vi "TraverseGetSetups.vi"(2 "Speed Factor":dbl=1.0 min=0.1 max=5.0 format="%.2f", 3 "Traverse Name":string="EnFlo Tunnel", 4 "Home":T2) -> (0 "Channel Properties Out":T1[](array[typedef]) {"Current Pos" format="%.2f"; "Backlash/Eng units" format="%.2f"; "Pulses/rev" format="%.2f"; "Pos Tolerance" format="%.2f"; "Pulses/unit" format="%.2f"; "Acc. Min" format="%.2f"; "Acc. Max" format="%.2f"; "Vel. Min" format="%.2f"; "Vel. Max" format="%.2f"; "Acc. Default" format="%.2f"; "Vel. Default" format="%.2f"}, 1 "Error String":string)   [LabVIEW 2022 SP3]
uses:
  Anemometry/Anemometry Sub Vis/Controls/Home.ctl
  ~subVIs/DriveConfigGlobal.vi
  ~subVIs/DriveProperties.ctl
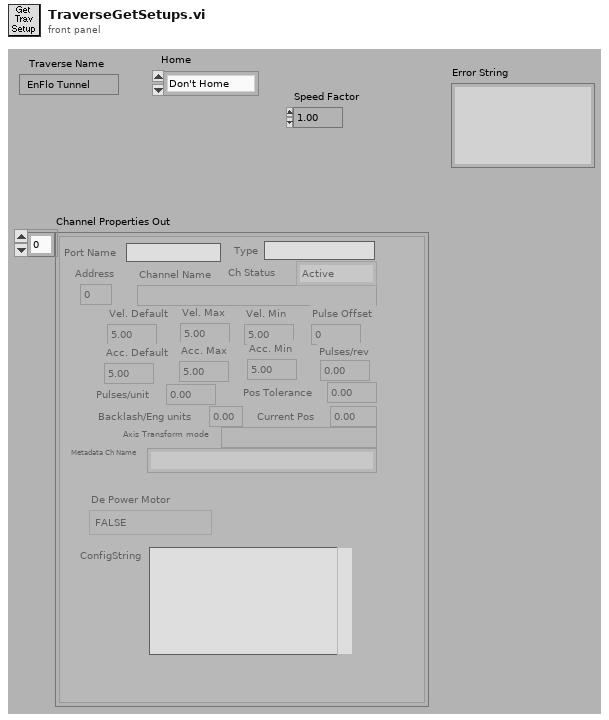
[diagram p1: front panel]
types:
  T1 = typedef "DriveProperties.ctl" = cluster{"Channel Name":string, "Vel. Default":sgl, "Acc. Default":sgl, "Vel. Max":sgl, "Vel. Min":sgl, "Acc. Max":sgl, "Acc. Min":sgl, "Pulses/unit":sgl, "Address":u8, "Pulse Offset":i32, "Pos Tolerance":sgl, "Pulses/rev":sgl, "Backlash/Eng units":sgl, "Current Pos":sgl, "Ch Status":enum16{"Active", "Offline", "Simulate"}, "Port Name":string, "Axis Transform mode":string, "Metadata Ch Name":string, "Type":string, "De Power Motor":enum16{"TRUE", "FALSE"}, "ConfigString":string}
  T2 = typedef "Home.ctl" = enum16{"Don't Home", "Home  +X", "Home  -X", "Home  +Y", "Home  -Y", "Home  +Z", "Home  -Z"}
  T3 = enum16{"Load setup from excel file", "Save setup to excel file"}
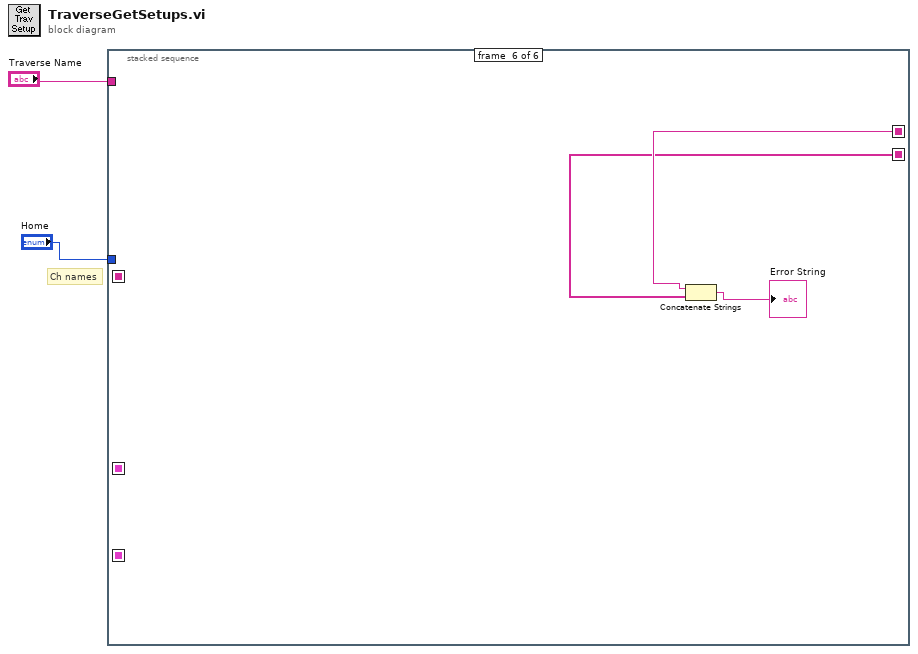
[diagram p0: block diagram]
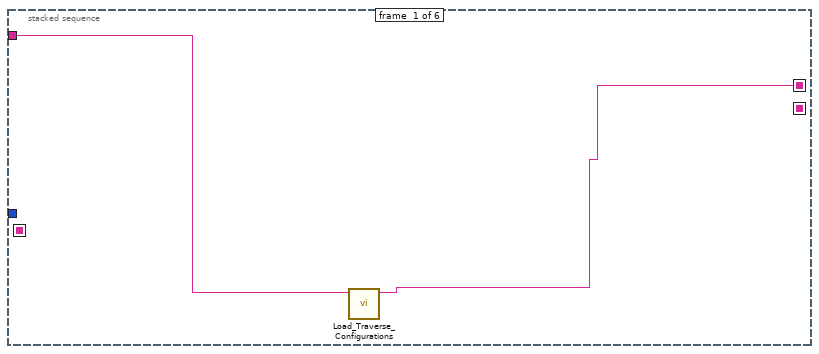
[diagram p2: hidden frame]
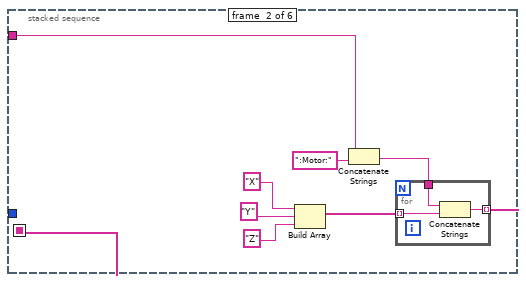
[diagram p3: hidden frame]
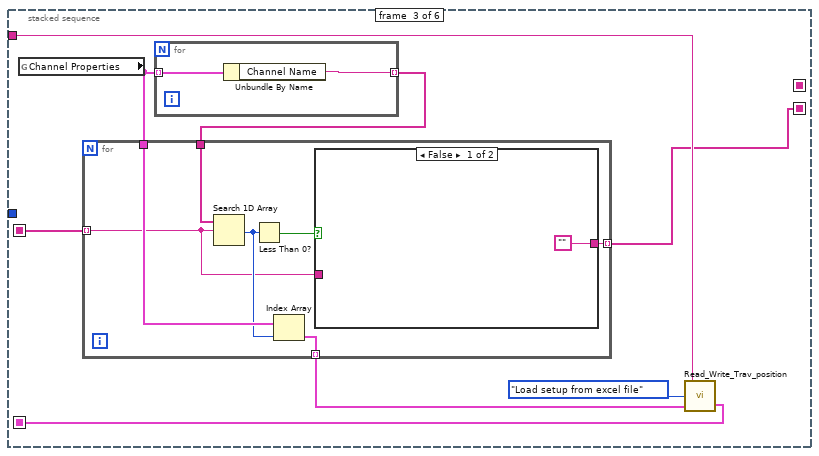
[diagram p4: hidden frame]
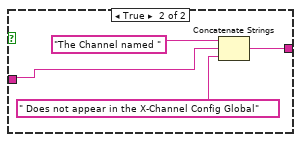
[diagram p5: hidden frame]
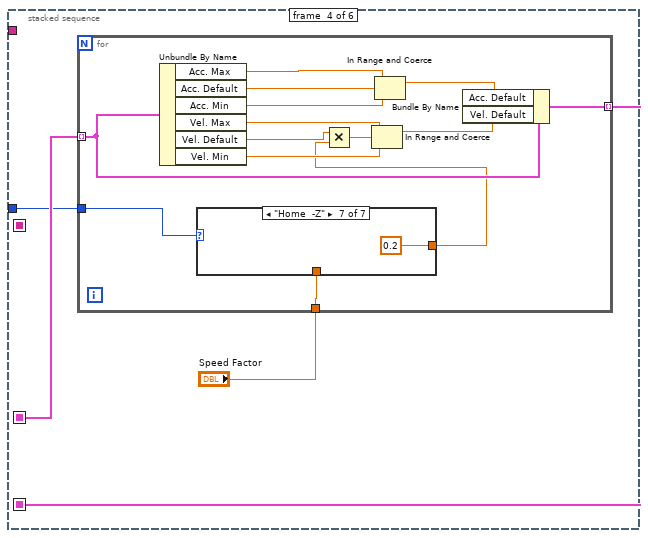
[diagram p6: hidden frame]
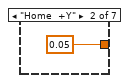
[diagram p8: hidden frame]
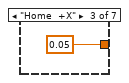
[diagram p9: hidden frame]
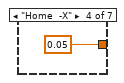
[diagram p10: hidden frame]
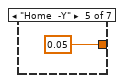
[diagram p11: hidden frame]
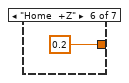
[diagram p12: hidden frame]
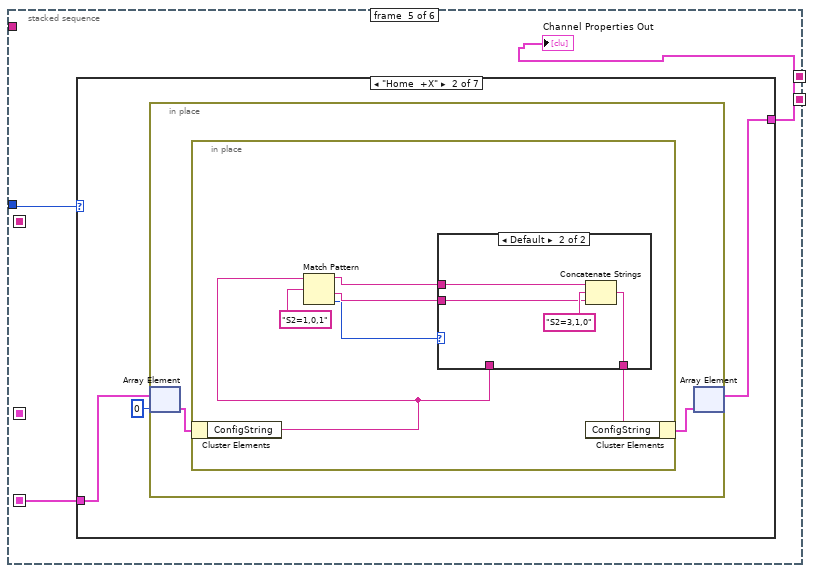
[diagram p13: hidden frame]
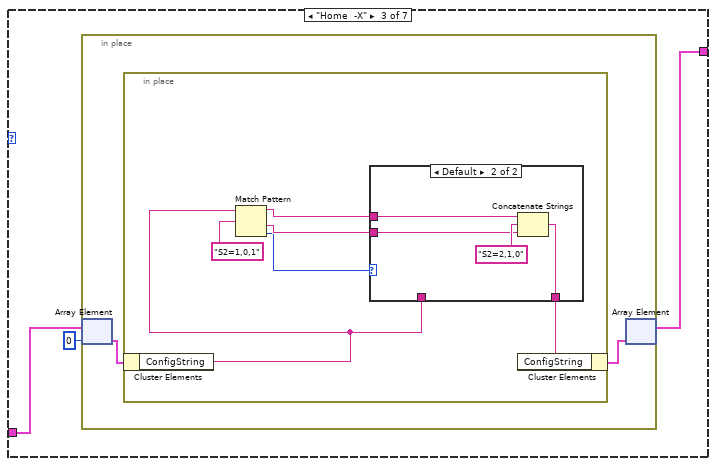
[diagram p16: hidden frame]
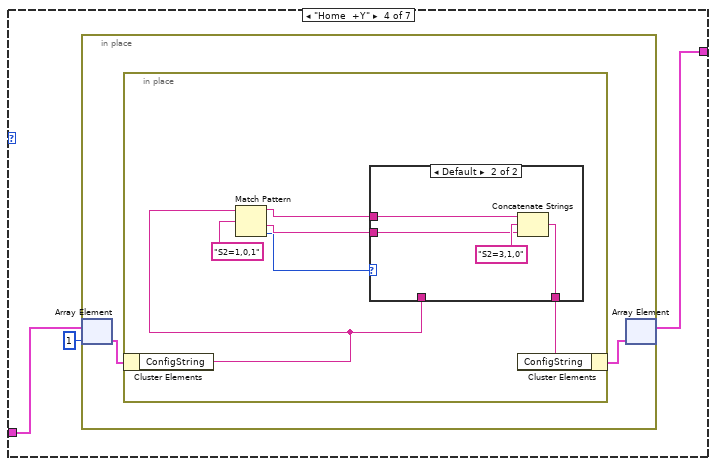
[diagram p18: hidden frame]
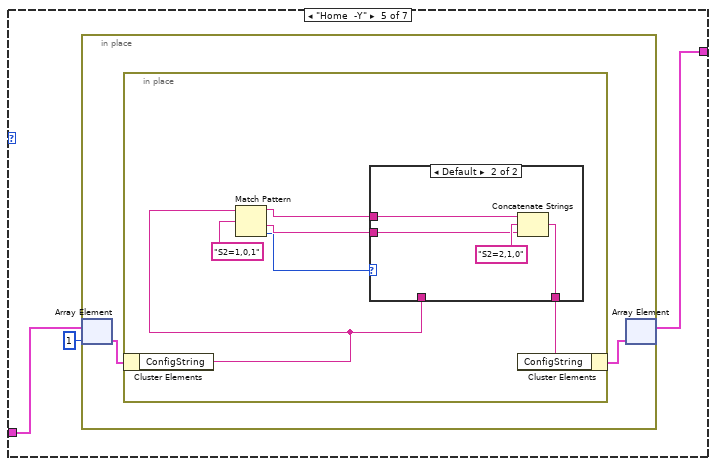
[diagram p20: hidden frame]
diagram:
  # "Ch names"
  n1 = stacked-sequence {
    seq-local: [_ w10 _ _ _ _] -> [_ _ w22 _ _ _]
    seq-local: [_ _ w19 _ _ _] -> [_ _ _ w41 _ _]
    seq-local: [_ _ _ w38 _ _] -> [_ _ _ _ w64 _]
    seq-local: [w3 _ _ _ _ _] -> [_ _ _ _ _ w165]
    seq-local: [_ _ w16 _ _ _] -> [_ _ _ _ _ w164]
    tunnel: "Traverse Name" -> [w4 w8 w18 _ _ _]
    tunnel: "Home" -> [_ _ _ w39 w65 _]
    frame #0 {
      n2 = call "Load_Traverse_Configurations.vi"("Traverse Name"=w4) -> ("Error String"=w3:string)  [unwired: 10 in]
    }
    frame #1 {
      n3 = Build Array("X", "Y", "Z") -> (w11:string[])
      n4 = Concatenate Strings(w8, ":Motor:") -> (w9:string)
      n5 = for {
        tunnel: w11 -> [w15] mode=indexing
        tunnel: [w13] -> w10 mode=indexing
        tunnel: w9 -> [w14]
        n6 = Concatenate Strings(w14, w15) -> (w13:string)
      }
    }
    frame #2 {
      n7 = global read "DriveConfigGlobal.vi" "Channel Properties"() -> (w17:T1[])
      n8 = for {
        tunnel: w17 -> [w37] mode=indexing
        tunnel: [w36] -> w23 mode=indexing
        n9 = Unbundle By Name(w37) -> ("Channel Name"=w36:string)
      }
      n10 = for {
        tunnel: w23 -> [w30]
        tunnel: w17 -> [w28]
        tunnel: [w26] -> w21 mode=indexing
        tunnel: w22 -> [w25] mode=indexing
        tunnel: [w24] -> w16 mode=indexing
        n11 = Search 1D Array(1D array=w30, element=w25) -> (index of element=w27:i32)  [unwired: 1 out]
        n12 = Less Than 0?(x=w27) -> (x < 0?=w29:bool)
        n13 = Index Array(array=w28, index=w27) -> (element=w26:T1)
        n14 = case shown="False" w29 {
          tunnel: w25 -> [_ w34]
          tunnel: ["" w32] -> w24
          frame False {
          }
          frame True {
            n15 = Concatenate Strings("The Channel named " ("message"), w34, " Does not appear in the X-Channel Config Global" ("Input 3")) -> (w32:string)
          }
        }
      }
      n16 = call "Read_Write_Trav_position.vi"("Channel Properties"=w21, "Mode"=T3."Load setup from excel file", "Traverse Name"=w18) -> ("Channel Properties Out"=w19:T1[])  [unwired: 1 out]
    }
    frame #3 {
      n17 = for {
        tunnel: w41 -> [w53] mode=indexing
        tunnel: "Speed Factor" -> [w45]
        tunnel: [w51] -> w38 mode=indexing
        tunnel: w39 -> [w43]
        n18 = Unbundle By Name(w53) -> ("Acc. Max"=w49:sgl, "Acc. Default"=w42:sgl, "Acc. Min"=w48:sgl, "Vel. Max"=w52:sgl, "Vel. Default"=w46:sgl, "Vel. Min"=w55:sgl)
        n19 = case shown="\"Home  -Z\"" w43 {
          tunnel: [w56 0.05 ("Speed Factor") 0.05 ("Speed Factor") 0.05 ("Speed Factor") 0.05 ("Speed Factor") 0.2 ("Speed Factor") 0.2 ("Speed Factor")] -> w44
          tunnel: w45 -> [w56 _ _ _ _ _ _]
          frame "Don't Home" {
          }
          frame "Home  +Y" {
          }
          frame "Home  +X" {
          }
          frame "Home  -X" {
          }
          frame "Home  -Y" {
          }
          frame "Home  +Z" {
          }
          frame "Home  -Z" {
          }
        }
        n20 = Multiply(x=w46, y=w44) -> (x*y=w54:dbl)
        n21 = In Range and Coerce(upper limit=w52, x=w54, lower limit=w55) -> (coerced(x)=w50:dbl)  [unwired: 1 out]
        n22 = In Range and Coerce(upper limit=w49, x=w42, lower limit=w48) -> (coerced(x)=w47:sgl)  [unwired: 1 out]
        n23 = Bundle By Name(cluster=w53, "Acc. Default"=w47, "Vel. Default"=w50) -> (w51:T1)
      }
    }
    frame #4 {
      n24 = case shown="\"Home  +X\"" w65 {
        tunnel: w64 -> [w66 w69 w85 w101 w117 w133 w149]
        tunnel: [w66 w67 w83 w99 w115 w131 w147] -> w63
        frame "Don't Home" {
        }
        frame "Home  +X" {
          n25 = in-place {
            n26 = in-place-array #1(w69, 0) -> (w71:T1)
            n27 = in-place {
              n28 = in-place-cluster #2(w71) -> ("ConfigString"=w72:string)
              n29 = Match Pattern(string=w72, regular expression="S2=1,0,1") -> (before substring=w76:string, after substring=w75:string, offset past match=w73:i32)  [unwired: 1 in, 1 out]
              n30 = case shown="Default" w73 {
                tunnel: w76 -> [_ w82]
                tunnel: w75 -> [_ w80]
                tunnel: [w78 w79] -> w74
                tunnel: w72 -> [w78 _]
                frame -1 {
                }
                frame Default {
                  n31 = Concatenate Strings(w82, "S2=3,1,0" ("regular expression"), w80) -> (w79:string)
                }
              }
              n32 = in-place-cluster #2("ConfigString"=w74) -> (w70:T1)
            }
            n33 = in-place-array #1(w70) -> (w67:T1[])  [unwired: 1 out]
          }
        }
        frame "Home  -X" {
          n34 = in-place {
            n35 = in-place-array #3(w85, 0) -> (w87:T1)
            n36 = in-place {
              n37 = in-place-cluster #4(w87) -> ("ConfigString"=w88:string)
              n38 = Match Pattern(string=w88, regular expression="S2=1,0,1") -> (before substring=w92:string, after substring=w91:string, offset past match=w89:i32)  [unwired: 1 in, 1 out]
              n39 = case shown="Default" w89 {
                tunnel: w92 -> [_ w98]
                tunnel: w91 -> [_ w96]
                tunnel: [w94 w95] -> w90
                tunnel: w88 -> [w94 _]
                frame -1 {
                }
                frame Default {
                  n40 = Concatenate Strings(w98, "S2=2,1,0" ("regular expression"), w96) -> (w95:string)
                }
              }
              n41 = in-place-cluster #4("ConfigString"=w90) -> (w86:T1)
            }
            n42 = in-place-array #3(w86) -> (w83:T1[])  [unwired: 1 out]
          }
        }
        frame "Home  +Y" {
          n43 = in-place {
            n44 = in-place-array #5(w101, 1) -> (w103:T1)
            n45 = in-place {
              n46 = in-place-cluster #6(w103) -> ("ConfigString"=w104:string)
              n47 = Match Pattern(string=w104, regular expression="S2=1,0,1") -> (before substring=w108:string, after substring=w107:string, offset past match=w105:i32)  [unwired: 1 in, 1 out]
              n48 = case shown="Default" w105 {
                tunnel: w108 -> [_ w114]
                tunnel: w107 -> [_ w112]
                tunnel: [w110 w111] -> w106
                tunnel: w104 -> [w110 _]
                frame -1 {
                }
                frame Default {
                  n49 = Concatenate Strings(w114, "S2=3,1,0" ("regular expression"), w112) -> (w111:string)
                }
              }
              n50 = in-place-cluster #6("ConfigString"=w106) -> (w102:T1)
            }
            n51 = in-place-array #5(w102) -> (w99:T1[])  [unwired: 1 out]
          }
        }
        frame "Home  -Y" {
          n52 = in-place {
            n53 = in-place-array #7(w117, 1) -> (w119:T1)
            n54 = in-place {
              n55 = in-place-cluster #8(w119) -> ("ConfigString"=w120:string)
              n56 = Match Pattern(string=w120, regular expression="S2=1,0,1") -> (before substring=w124:string, after substring=w123:string, offset past match=w121:i32)  [unwired: 1 in, 1 out]
              n57 = case shown="Default" w121 {
                tunnel: w124 -> [_ w130]
                tunnel: w123 -> [_ w128]
                tunnel: [w126 w127] -> w122
                tunnel: w120 -> [w126 _]
                frame -1 {
                }
                frame Default {
                  n58 = Concatenate Strings(w130, "S2=2,1,0" ("regular expression"), w128) -> (w127:string)
                }
              }
              n59 = in-place-cluster #8("ConfigString"=w122) -> (w118:T1)
            }
            n60 = in-place-array #7(w118) -> (w115:T1[])  [unwired: 1 out]
          }
        }
        frame "Home  +Z" {
          n61 = in-place {
            n62 = in-place-array #9(w133, 2) -> (w135:T1)
            n63 = in-place {
              n64 = in-place-cluster #10(w135) -> ("ConfigString"=w136:string)
              n65 = Match Pattern(string=w136, regular expression="S2=1,0,1") -> (before substring=w140:string, after substring=w139:string, offset past match=w137:i32)  [unwired: 1 in, 1 out]
              n66 = case shown="Default" w137 {
                tunnel: w140 -> [_ w146]
                tunnel: w139 -> [_ w144]
                tunnel: [w142 w143] -> w138
                tunnel: w136 -> [w142 _]
                frame -1 {
                }
                frame Default {
                  n67 = Concatenate Strings(w146, "S2=3,1,0" ("regular expression"), w144) -> (w143:string)
                }
              }
              n68 = in-place-cluster #10("ConfigString"=w138) -> (w134:T1)
            }
            n69 = in-place-array #9(w134) -> (w131:T1[])  [unwired: 1 out]
          }
        }
        frame "Home  -Z" {
          n70 = in-place {
            n71 = in-place-array #11(w149, 2) -> (w151:T1)
            n72 = in-place {
              n73 = in-place-cluster #12(w151) -> ("ConfigString"=w152:string)
              n74 = Match Pattern(string=w152, regular expression="S2=1,0,1") -> (before substring=w156:string, after substring=w155:string, offset past match=w153:i32)  [unwired: 1 in, 1 out]
              n75 = case shown="Default" w153 {
                tunnel: w156 -> [_ w162]
                tunnel: w155 -> [_ w160]
                tunnel: [w158 w159] -> w154
                tunnel: w152 -> [w158 _]
                frame -1 {
                }
                frame Default {
                  n76 = Concatenate Strings(w162, "S2=3,1,0" ("regular expression"), w160) -> (w159:string)
                }
              }
              n77 = in-place-cluster #12("ConfigString"=w154) -> (w150:T1)
            }
            n78 = in-place-array #11(w150) -> (w147:T1[])  [unwired: 1 out]
          }
        }
      }
      "Channel Properties Out" <- w63
    }
    frame #5 {
      n79 = Concatenate Strings(w165, w164) -> (→"Error String":string)
    }
  }
